vi "Launch Command Helper.vi"(7 "Description":string, 8 "Command Info In":T3, 11 "SubSystem Data":T1) -> (0 "Command Info Out":T3, 3 "SubSystem Data":T1)   [LabVIEW 2016]
uses:
  Launch Setpoints.ctl
  Launch Operations.ctl
  <vilib>/Rock Robotics/WPI/Framework/Command Status Info.ctl
  <vilib>/Rock Robotics/WPI/Framework/Completion Status.ctl
  <vilib>/Rock Robotics/WPI/Framework/Completion Notifier.ctl
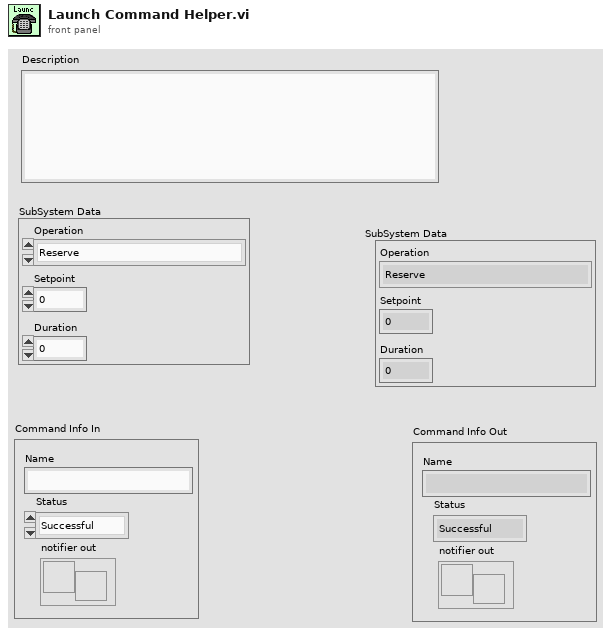
[diagram p1: front panel]
types:
  T1 = typedef "Launch Setpoints.ctl" = cluster{"Operation":T2, "Setpoint":dbl, "Duration":dbl}
  T2 = typedef "Launch Operations.ctl" = enum16{"Reserve", "Read Current", "Immediate", "Set Adgitator"}
  T3 = typedef "Command Status Info.ctl" = cluster{"Name":string, "Status":T4, "notifier out":T5}
  T4 = typedef "Completion Status.ctl" = enum16{"Successful", "Aborted", "Incomplete"}
  T5 = typedef "Completion Notifier.ctl" = refnum<notifier>
  T6 = cluster{"SubSystem Data":T1, "Command Info In":T3, string}
  T7 = cluster{"SubSystem Data":T1, "Command Info In":T3, "Description":string}
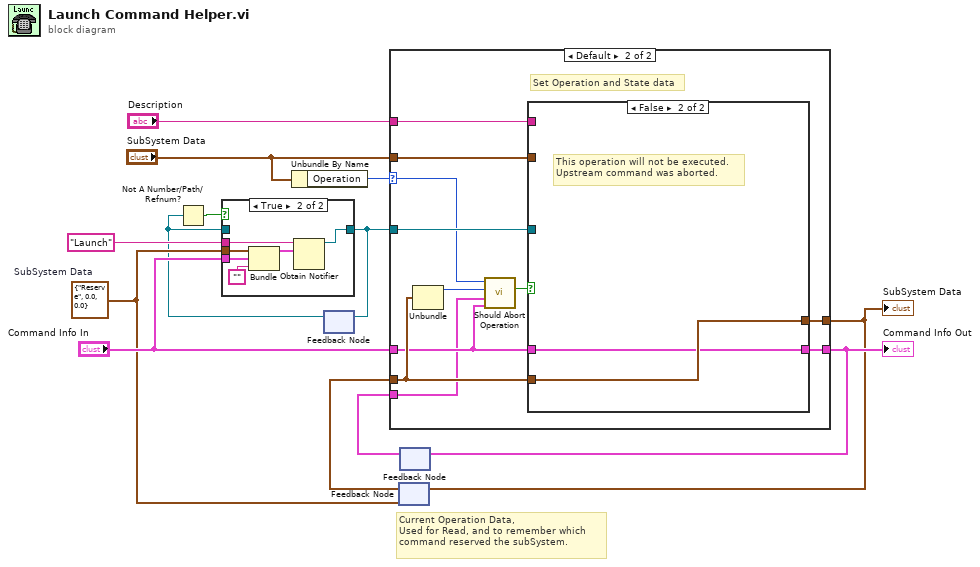
[diagram p0: block diagram]
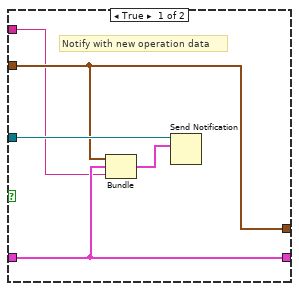
[diagram p4: hidden frame]
diagram:
  w5 = T1 {"Operation"=enum."Reserve", "Setpoint"=0.0, "Duration"=0.0}  # SubSystem Data
  # "Current Operation Data,\nUsed for Read, and to remember which\ncommand reserved the subSystem."
  n1 = Unbundle By Name("SubSystem Data") -> ("Operation"=w11:T2)
  n2 = feedback #1() -> (w2:refnum<notifier>)  [unwired: 1 in]
  n3 = Not A Number/Path/Refnum?(number/path/refnum=w2) -> (NaN/Path/Refnum?=w3:bool)
  n4 = case shown="True" w3 {
    tunnel: "Launch" -> [_ w20]
    tunnel: [w14 w19] -> w9
    tunnel: w5 -> [_ w18]
    tunnel: "Command Info In" -> [_ w16]
    tunnel: w2 -> [w14 _]
    frame False {
    }
    frame True {
      n5 = Bundle("SubSystem Data"=w18, "Command Info In"=w16, "") -> (w17:T6)  [unwired: 1 in]
      n6 = Obtain Notifier(name (unnamed)=w20, notification data type=w17) -> (notifier out=w19:refnum<notifier>)  [unwired: 2 in, 2 out]
    }
  }
  n7 = feedback-in #1(w9) -> ()
  n8 = feedback #2(w5) -> (w13:T1)
  n9 = feedback #3() -> (w7:T3)  [unwired: 1 in]
  n10 = case shown="Default" w11 {
    selector: w11 -> [_ w28]
    tunnel: [w22 w30] -> w4
    tunnel: w9 -> [_ w32]
    tunnel: "SubSystem Data" -> [_ w33]
    tunnel: w13 -> [w22 w27]
    tunnel: [w21 w31] -> w8
    tunnel: "Command Info In" -> [_ w25]
    tunnel: w7 -> [w21 w24]
    tunnel: "Description" -> [_ w23]
    frame "Read Current" {
    }
    frame Default {
      # "Set Operation and State data"
      n11 = Unbundle(w27) -> ("Operation"=w26:T2)  [unwired: 2 out]
      n12 = call <vilib>:"Should Abort Operation.vi"("New Command Info"=w25, "Current Command Info"=w24, "Operation"=w26, "New Operation"=w28) -> ("Execute"=w29:bool)  [unwired: 7 in]
      n13 = case shown="False" w29 {
        tunnel: [w37 w40] -> w30
        tunnel: w33 -> [w37 _]
        tunnel: w32 -> [w38 _]
        tunnel: w27 -> [_ w40]
        tunnel: [w36 w39] -> w31
        tunnel: w25 -> [w36 w39]
        tunnel: w23 -> [w34 _]
        frame True {
          # "Notify with new operation data"
          n14 = Bundle("SubSystem Data"=w37, "Command Info In"=w36, "Description"=w34) -> (w35:T7)  [unwired: 1 in]
          n15 = Send Notification(notification=w35, notifier=w38) -> ()  [unwired: 1 in, 2 out]
        }
        frame False {
          # "This operation will not be executed.\nUpstream command was aborted."
        }
      }
    }
  }
  "Command Info Out" <- w8
  "SubSystem Data" <- w4
  n16 = feedback-in #2(w4) -> ()
  n17 = feedback-in #3(w8) -> ()
